vi "connect udp image server.vi"(1 "ImageServer":cluster{"IPAddress":string, "Port":i32}) -> (2 "connection ID":refnum<k16>, 4 "error out":errorcluster)   [LabVIEW 2013]
uses:
  <vilib>/Utility/tcp.llb/UDP Multicast Read-Only Open.vi
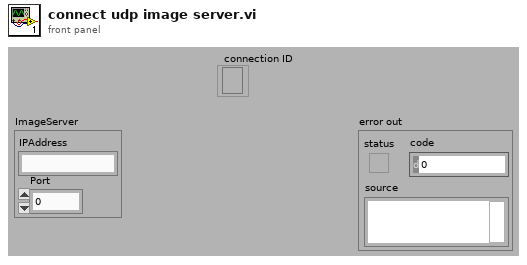
[diagram p1: front panel]
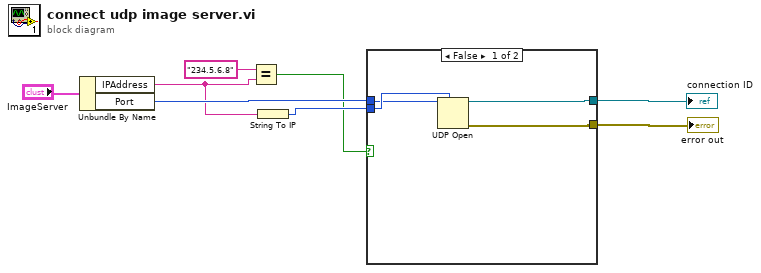
[diagram p0: block diagram]
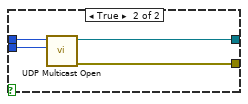
[diagram p2: hidden frame]
diagram:
  n1 = Unbundle By Name("ImageServer") -> ("IPAddress"=w3:string, "Port"=w8:i32)
  n2 = Equal?(x="234.5.6.8", y=w3) -> (x = y?=w1:bool)
  n3 = String To IP(1:w3) -> (0:w5:u32)
  n4 = case shown="False" w1 {
    tunnel: w8 -> [w9 w16]
    tunnel: [w10 w15] -> w7
    tunnel: w5 -> [w12 w14]
    tunnel: [w11 w13] -> w4
    frame False {
      n5 = UDP Open(7:w12, 11:w9) -> (port=w11:refnum<k16>, 0:w10:errorcluster)  [unwired: 3 in, 1 out]
    }
    frame True {
      n6 = call-poly <vilib>:"UDP Multicast Open.vi"("multicast addr"=w14, "port"=w16) -> ("error out"=w15:errorcluster, "connection ID"=w13:refnum<k16>)  [unwired: 2 in, 6 out]
    }
  }
  "error out" <- w7
  "connection ID" <- w4
